vi "20211029_01.vi"() -> ()   [LabVIEW 2019]
panel:
  in  "Enum":enum16{"1", "2", "3", "4", "5"}(ring)
  in  "Select":enum16{"1", "2", "3", "4", "5"}(ring)
  in  "Enable":bool
  in  "Disable":bool
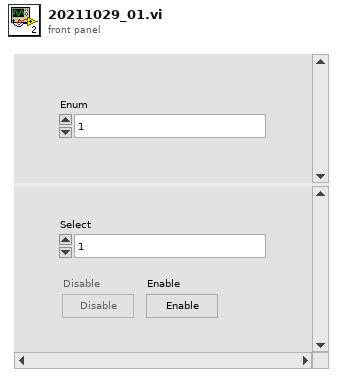
[diagram p1: front panel]
types:
  T1 = enum8{"Enabled", "Disabled", "Disabled and Grayed Out"}
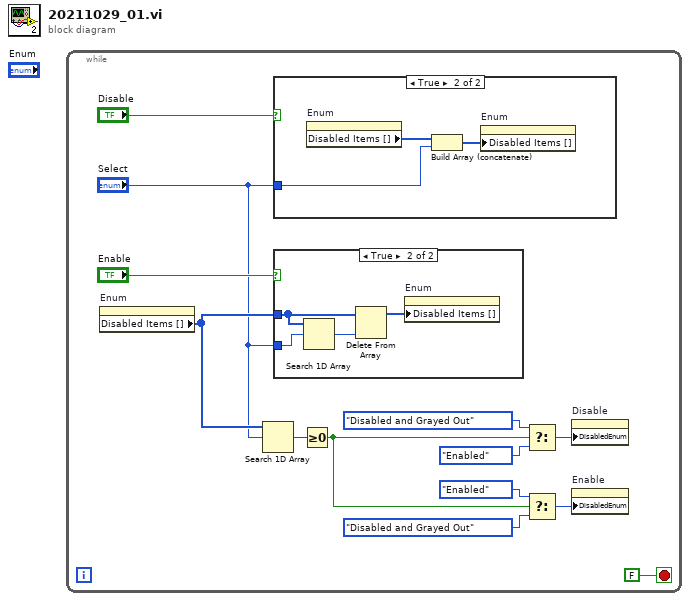
[diagram p0: block diagram]
diagram:
  n1 = while {
    stop <- FALSE stop-if-true
    n2 = property on="Enum" class="Enum (strict)"() -> ("Disabled Items []"=w10:i32[])  [unwired: 2 in, 2 out]
    n3 = Search 1D Array(1D array=w10, element="Select") -> (index of element=w8:i32)  [unwired: 1 in]
    n4 = case shown="True" "Disable" {
      tunnel: "Select" -> [_ w19]
      frame False {
      }
      frame True {
        n5 = property on="Enum" class="Enum (strict)"() -> ("Disabled Items []"=w20:i32[])  [unwired: 2 in, 2 out]
        n6 = Build Array (concatenate)(w20, w19) -> (w18:i32[])
        n7 = property on="Enum" class="Enum (strict)"("Disabled Items []"=w18) -> ()  [unwired: 2 in, 2 out]
      }
    }
    n8 = case shown="True" "Enable" {
      tunnel: "Select" -> [_ w17]
      tunnel: w10 -> [_ w14]
      frame False {
      }
      frame True {
        n9 = Search 1D Array(1D array=w14, element=w17) -> (index of element=w15:i32)  [unwired: 1 in]
        n10 = Delete From Array(array=w14, index=w15) -> (array with subset deleted=w16:i32[])  [unwired: 1 in, 1 out]
        n11 = property on="Enum" class="Enum (strict)"("Disabled Items []"=w16) -> ()  [unwired: 2 in, 2 out]
      }
    }
    n12 = Greater Or Equal To 0?(x=w8) -> (x >= 0?=w1:bool)
    n13 = Select(t=T1."Disabled and Grayed Out" ("Disabled"), s=w1, f=T1."Enabled" ("Disabled")) -> (s? t:f=w5:T1)
    n14 = Select(t=T1."Enabled" ("Disabled"), s=w1, f=T1."Disabled and Grayed Out" ("Disabled")) -> (s? t:f=w2:T1)
    n15 = property on="Disable" class="Bool"("DisabledEnum"=w5) -> ()  [unwired: 2 in, 2 out]
    n16 = property on="Enable" class="Bool"("DisabledEnum"=w2) -> ()  [unwired: 2 in, 2 out]
  }
